vi "test Get Base 8_2.vi"(11 "Test Case In":refnum<class "test Electronic Datasheet.lvclass">) -> (0 "error out":errorcluster, 3 "Test Case Out":refnum<class "test Electronic Datasheet.lvclass">)   [LabVIEW 2024, in "Test Utilities.lvclass"]
uses:
  Test Utilities.lvclass
  Test Utilities.lvclass/Test Utilities.ctl
  EDS-File-Viewer/Tests/source/test Electronic Datasheet/test Electronic Datasheet.lvclass
  <vilib>/Astemes/LUnit/Test Case.lvclass
  source/CANopen.lvlib
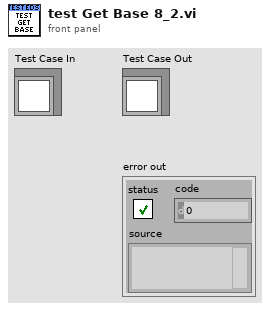
[diagram p1: front panel]
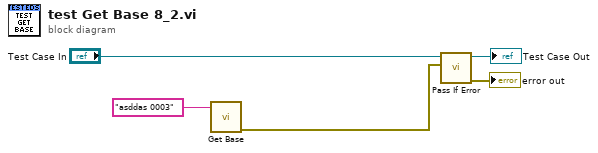
[diagram p0: block diagram]
diagram:
  n1 = call "Get Base.vi"("Default Value"="asddas 0003") -> ("error out"=w1:errorcluster)  [unwired: 8 in, 2 out]
  n2 = call <vilib>:"Pass If Error.vi"("Assert error"=w1, "LUnit Test Case In"="Test Case In") -> ("error out"=→"error out":errorcluster, "LUnit Test Case Out"=→"Test Case Out":refnum<class "test Electronic Datasheet.lvclass">)  [unwired: 8 in]
